vi "Cluster_example.vi"() -> ()   [LabVIEW 2019]
panel:
  out "output cluster":T1
  out "Gender 2":enum16{"", "Male", "Female", "Others"}(ring)
  in  "Gender":enum16{"", "Male", "Female", "Others"}(ring)=enum."Male"
  out "Salary 3":dbl
  out "Age 3":dbl
  out "Name 3":string
  in  "Salary":dbl=900000.0
  in  "Age":dbl=21.0
  in  "Name":string="Atharva"
  in  "Employee":T1
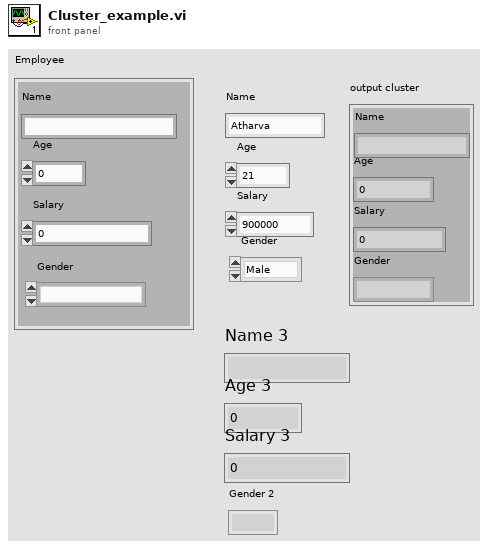
[diagram p1: front panel]
types:
  T1 = cluster{"Name":string, "Age":dbl, "Salary":dbl, "Gender":enum16{"", "Male", "Female", "Others"}}
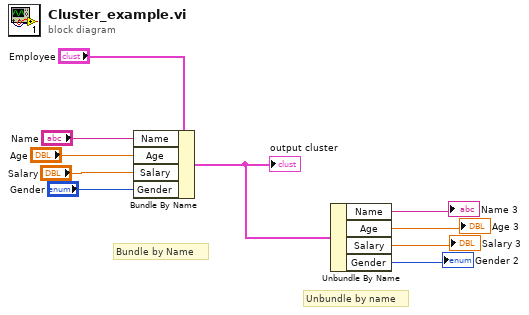
[diagram p0: block diagram]
diagram:
  # "Unbundle by name"
  # "Bundle by Name"
  n1 = Bundle By Name(cluster="Employee", "Name"="Name", "Age"="Age", "Salary"="Salary", "Gender"="Gender") -> (w1:T1)
  "output cluster" <- w1
  n2 = Unbundle By Name(w1) -> ("Name"=→"Name 3":string, "Age"=→"Age 3":dbl, "Salary"=→"Salary 3":dbl, "Gender"=→"Gender 2":enum16{"", "Male", "Female", "Others"})
